vi "get_external_stop.vi"(8 "stop_internal":bool, 11 "ref_stop_external":refnum<vi>) -> (3 "stop_output":bool)   [LabVIEW 2019]
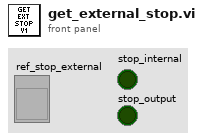
[diagram p1: front panel]
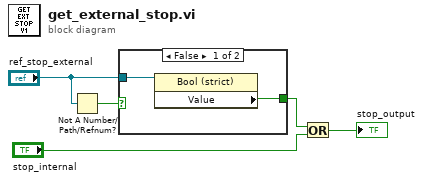
[diagram p0: block diagram]
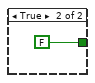
[diagram p2: hidden frame]
diagram:
  n1 = Not A Number/Path/Refnum?(number/path/refnum="ref_stop_external") -> (NaN/Path/Refnum?=w4:bool)
  n2 = case shown="False" w4 {
    tunnel: [w6 FALSE] -> w3
    tunnel: "ref_stop_external" -> [w7 _]
    frame False {
      n3 = property class="Bool (strict)"(reference=w7) -> ("Value"=w6:bool)  [unwired: 1 in, 2 out]
    }
    frame True {
    }
  }
  n4 = Or(x=w3, y="stop_internal") -> (x .or. y?=→"stop_output":bool)
